vi "Initialize.vi"(8 "error in (no error)":errorcluster, 9 "Components":refnum<class "Component.lvclass">[](array[class]), 10 "plugin configuration":T3, 11 "Plugin Configuration in":refnum<class "Plugin Configuration.lvclass">) -> (0 "error out":errorcluster, 3 "Plugin Configuration out":refnum<class "Plugin Configuration.lvclass">)   [LabVIEW 2017, in "DSF Core.lvlib" / "Plugin Configuration.lvclass"]
uses:
  Plugin Configuration.lvclass
  Typedefs/DSF Component Configuration.ctl
  Typedefs/DSF Version Info.ctl
  Component/Component.lvclass
  Core/Plugin/Core Plugins Configuration.lvclass
  Plugin Configuration.lvclass/Plugin Configuration.ctl
  Configuration.lvclass
  Thread/Thread Configuration.lvclass
  DSF Core.lvlib
  Component Configuration/Component Configuration.lvclass
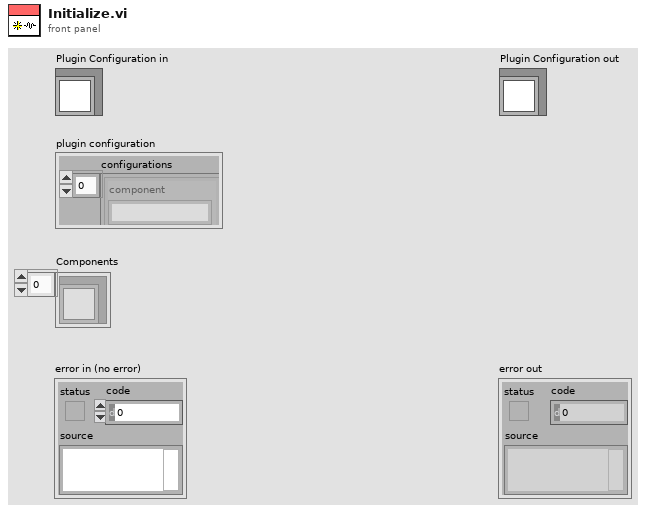
[diagram p1: front panel]
types:
  T1 = typedef "DSF Core.lvlib/DSF Component Configuration.ctl" = cluster{"component":string, "data":string, "data version":T2}
  T2 = typedef "DSF Core.lvlib/DSF Version Info.ctl" = cluster{"major":i32, "minor":i32, "fix":i32, "build":string}
  T3 = cluster{"configurations":T1[], "threads":cluster{"configurations":T1[], "groups":cluster{"configurations":T1[], "transfers":cluster{"configurations":T1[]}[]}[]}[]}
  T4 = cluster{"configurations":T1[], "groups":cluster{"configurations":T1[], "transfers":cluster{"configurations":T1[]}[]}[]}[]
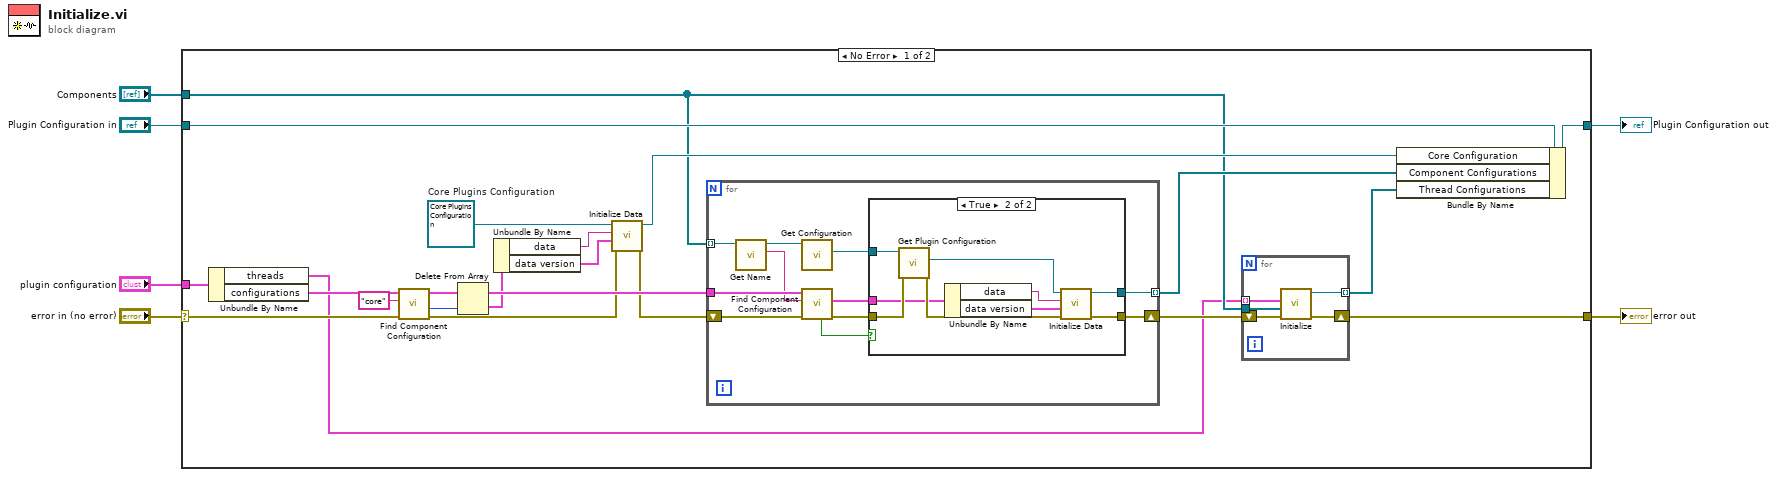
[diagram p0: block diagram]
diagram:
  n1 = case shown="No Error" "error in (no error)" {
    selector: "error in (no error)" -> [w8 w56]
    tunnel: "plugin configuration" -> [w28 _]
    tunnel: "Plugin Configuration in" -> [w16 w55]
    tunnel: [w15 w55] -> w4
    tunnel: [w10 w56] -> w3
    tunnel: "Components" -> [w9 _]
    frame No Error {
      w22 = refnum<class "Core Plugins Configuration.lvclass"> refnum  # Core Plugins Configuration
      n2 = Unbundle By Name(w28) -> ("threads"=w7:T4, "configurations"=w26:T1[])
      n3 = call "Find Component Configuration.vi"("error in (no error)"=w8, "component"="core", "configurations in"=w26) -> ("error out"=w20:errorcluster, "index"=w24:i32, "configurations out"=w25:T1[])  [unwired: 4 in, 2 out]
      n4 = Delete From Array(array=w25, index=w24) -> (deleted portion=w21:T1, array with subset deleted=w23:T1[])  [unwired: 1 in]
      n5 = Unbundle By Name(w21) -> ("data"=w18:string, "data version"=w17:T2)
      n6 = call-dynamic "Initialize Data.vi"("error in (no error)"=w20, "data version"=w17, "data"=w18, "Core Plugins Configuration in"=w22) -> ("error out"=w19:errorcluster, "Core Plugins Configuration out"=w14:refnum<class "Core Plugins Configuration.lvclass">)  [unwired: 6 in]
      n7 = for {
        tunnel: w9 -> [w33] mode=indexing
        tunnel: w23 -> [w35]
        shift-right: [w37] -> w12
        shift-left: w19 -> [w31]
        tunnel: [w34] -> w13 mode=indexing
        n8 = call "Get Name.vi"("Component in"=w33) -> ("name"=w32:string, "Component out"=w30:refnum<class "Component.lvclass">)  [unwired: 9 in]
        n9 = call "Get Configuration.vi"("Component in"=w30) -> ("Configuration"=w29:refnum<class "Component Configuration.lvclass">)  [unwired: 9 in, 1 out]
        n10 = call "Find Component Configuration.vi"("error in (no error)"=w31, "component"=w32, "configurations in"=w35) -> ("error out"=w38:errorcluster, "component configuration"=w36:T1, "found?"=w39:bool)  [unwired: 4 in, 2 out]
        n11 = case shown="True" w39 {
          tunnel: w38 -> [w40 w49]
          tunnel: [w40 w48] -> w37
          tunnel: w36 -> [_ w45]
          tunnel: [_ w42] -> w34
          tunnel: w29 -> [_ w41]
          frame False {
          }
          frame True {
            n12 = call "Get Plugin Configuration.vi"("error in (no error)"=w49, "Component Configuration in"=w41) -> ("error out"=w47:errorcluster, "Plugin Configuration"=w46:refnum<class "Configuration.lvclass">)  [unwired: 7 in, 1 out]
            n13 = Unbundle By Name(w45) -> ("data"=w44:string, "data version"=w43:T2)
            n14 = call-dynamic "Initialize Data.vi"("error in (no error)"=w47, "data version"=w43, "data"=w44, "Configuration in"=w46) -> ("error out"=w48:errorcluster, "Configuration out"=w42:refnum<class "Configuration.lvclass">)  [unwired: 6 in]
          }
        }
      }
      n15 = for {
        tunnel: [w53] -> w11 mode=indexing
        shift-right: [w52] -> w10
        shift-left: w12 -> [w54]
        tunnel: w9 -> [w50]
        tunnel: w7 -> [w51] mode=indexing
        n16 = call "Initialize.vi"("error in (no error)"=w54, "Components"=w50, "thread configuration"=w51) -> ("error out"=w52:errorcluster, "Thread Configuration out"=w53:refnum<class "Thread Configuration.lvclass">)  [unwired: 7 in]
      }
      n17 = Bundle By Name(cluster=w16, "Core Configuration"=w14, "Component Configurations"=w13, "Thread Configurations"=w11) -> (w15:refnum<class "Plugin Configuration.lvclass">)
    }
    frame Error {
    }
  }
  "error out" <- w3
  "Plugin Configuration out" <- w4
